vi "Fetch Device Info.vi"(8 "error in (no error)":errorcluster, 11 "Toggle 8 in":refnum<class "Toggle 8.lvclass">) -> (0 "error out":errorcluster, 2 "Device Info":string[][](array[string]), 3 "Toggle 8 out":refnum<class "Toggle 8.lvclass">)   [LabVIEW 2020, in "Toggle 8.lvclass"]
uses:
  Toggle 8.lvclass
  PIC-device/PIC-Device.lvclass
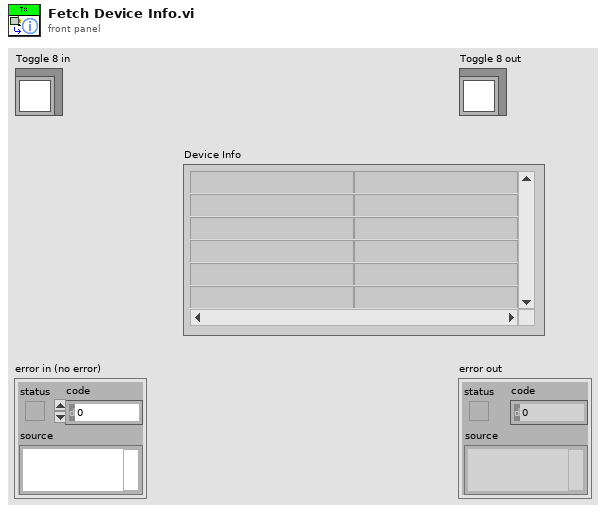
[diagram p1: front panel]
types:
  T1 = typedef "PIC-Device.lvclass/Register to Write.ctl" = cluster{"Register":u32, "Value":u32, "Dev Address":u32, "Physical Adress":u32}
  T2 = typedef "Device.lvclass/Device Information Cluster.ctl" = cluster{"Device Info":string[][], "Default Values":T1[], "Fetched info":string[][]}
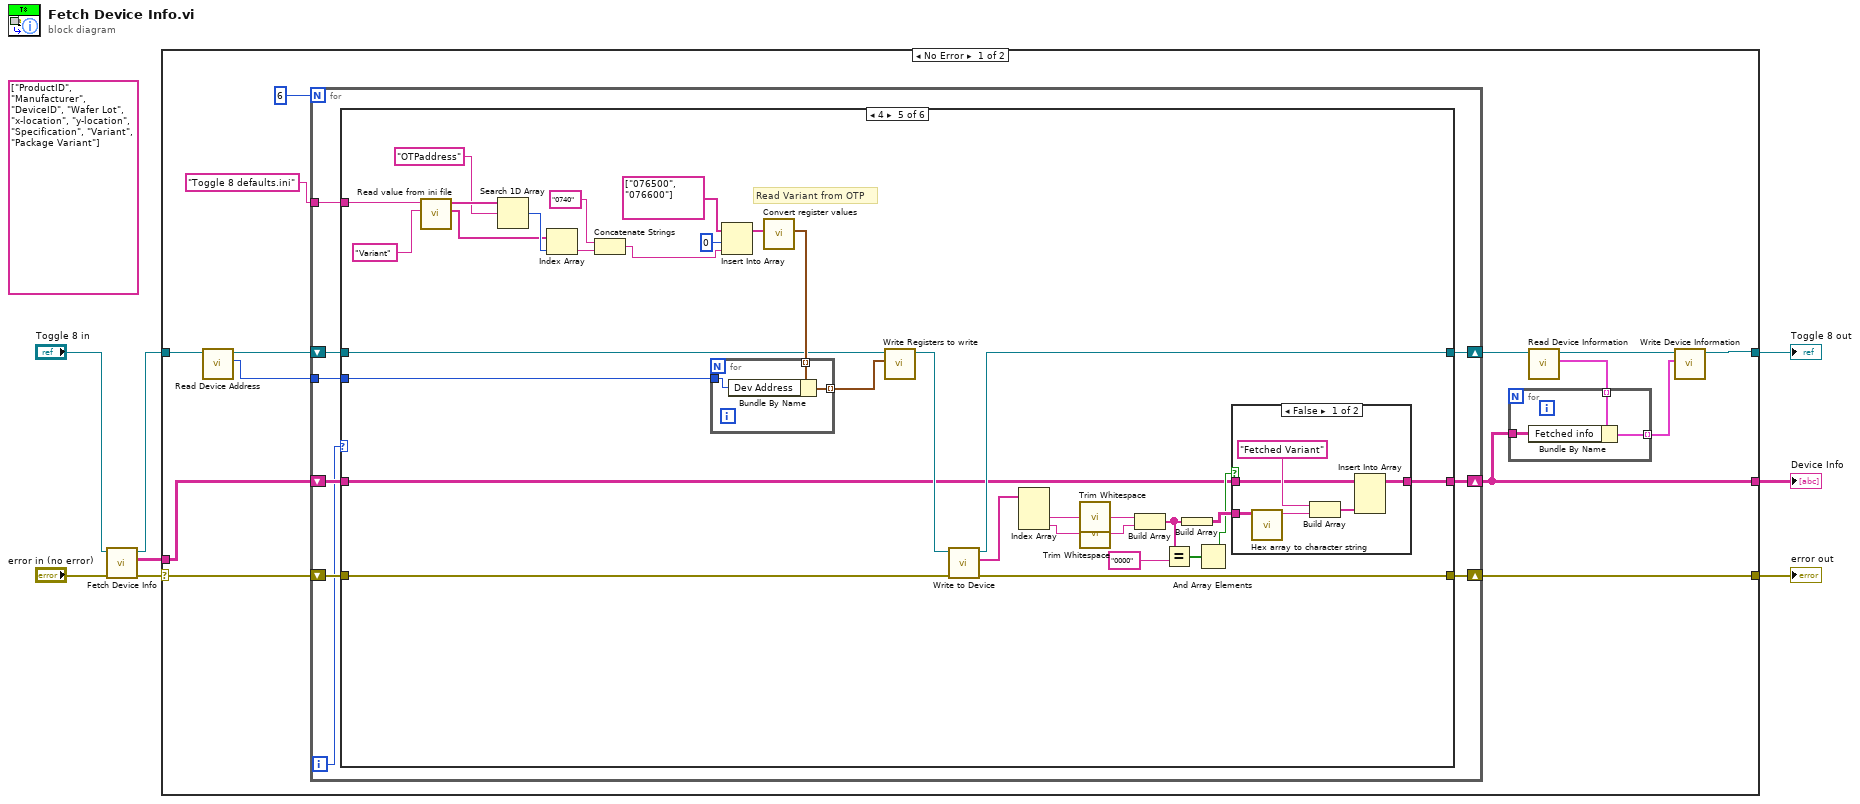
[diagram p0: block diagram]
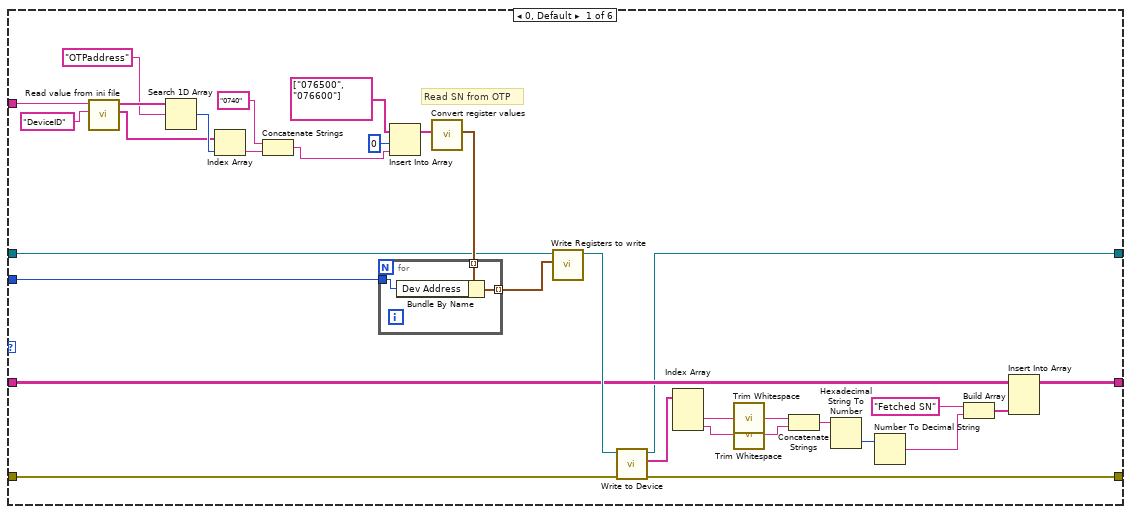
[diagram p2: hidden frame]
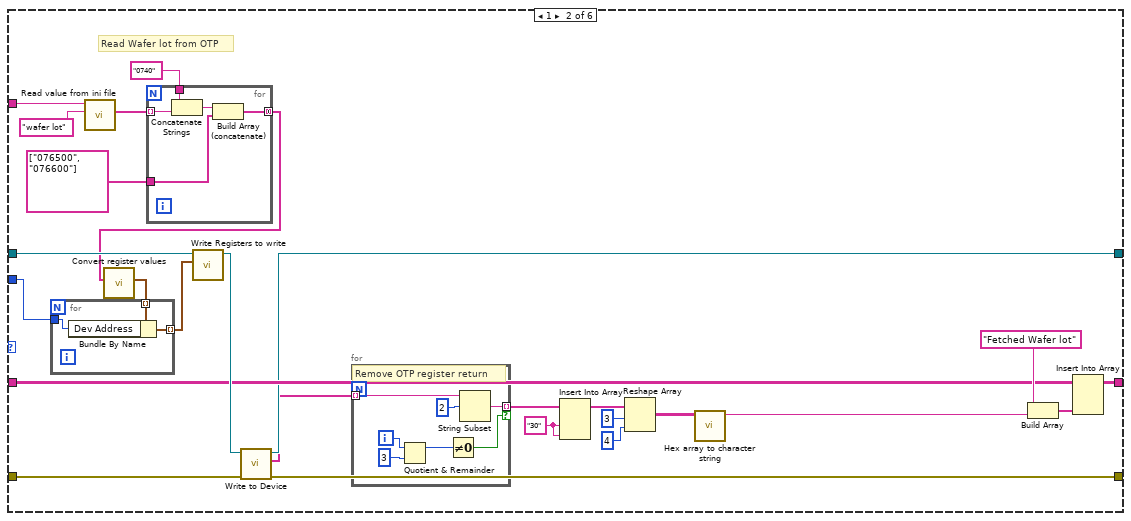
[diagram p3: hidden frame]
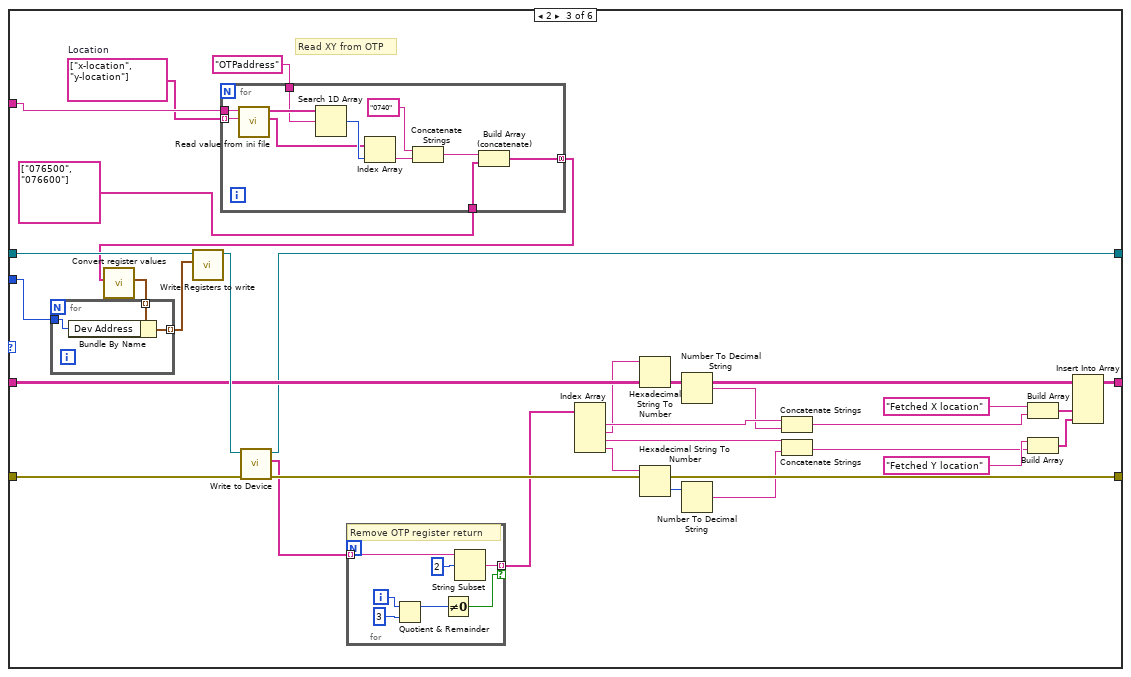
[diagram p4: hidden frame]
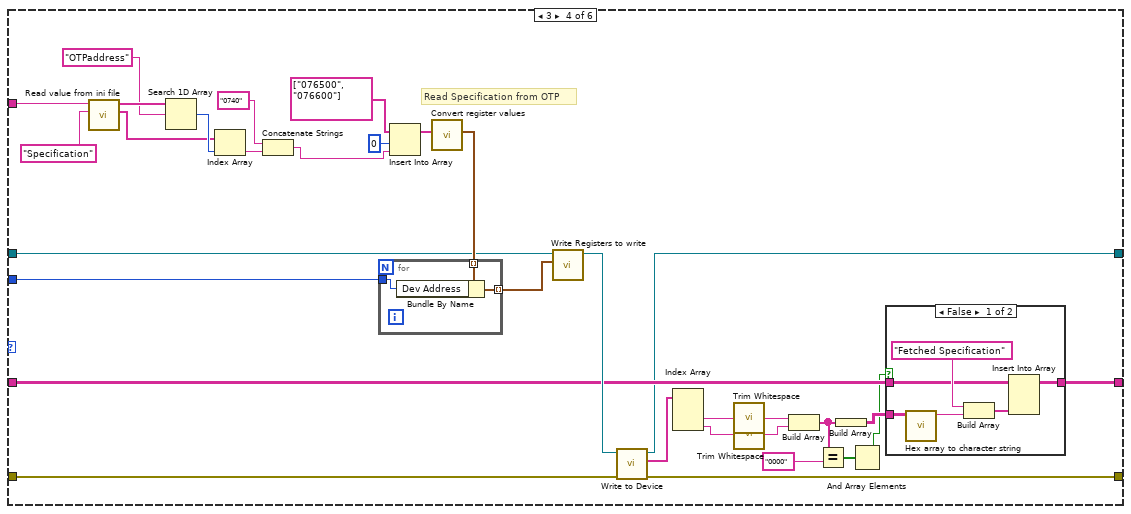
[diagram p5: hidden frame]
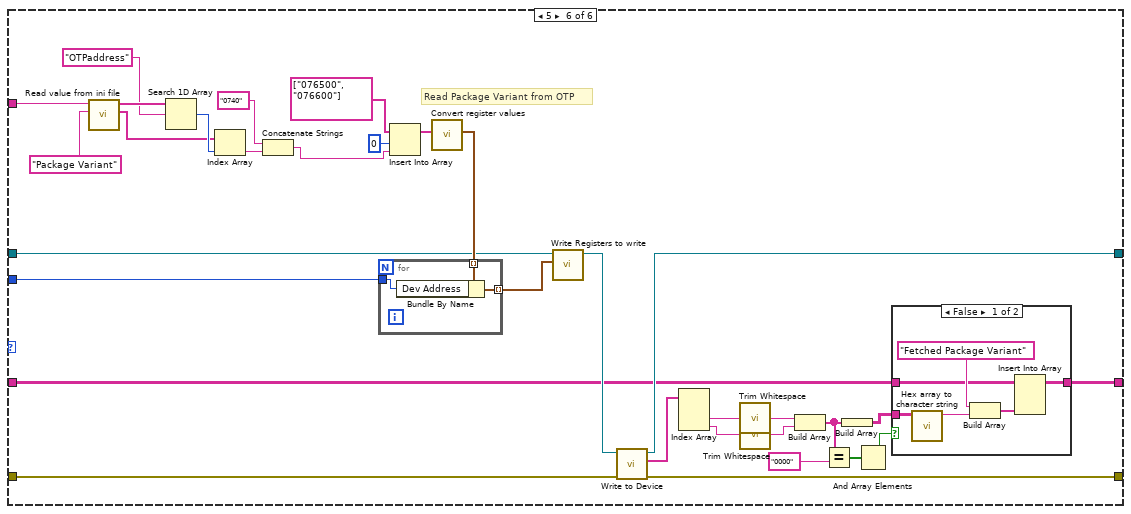
[diagram p8: hidden frame]
diagram:
  (unwired) string[] ["ProductID", "Manufacturer", "DeviceID", "Wafer Lot", "x-location", "y-location", "Specification", "Variant", "Package Variant"]
  n1 = call-parent "Fetch Device Info.vi"("error in (no error)"="error in (no error)", "PIC-Device in"="Toggle 8 in") -> ("error out"=w5:errorcluster, "Device Info"=w2:string[][], "PIC-Device out"=w3:refnum<class "Toggle 8.lvclass">)  [unwired: 7 in]
  n2 = case shown="No Error" w5 {
    selector: w5 -> [w22 w291]
    tunnel: [w20 w291] -> w8
    tunnel: [w14 w290] -> w7
    tunnel: w3 -> [w19 w290]
    tunnel: w2 -> [w21 w289]
    tunnel: [w13 w289] -> w1
    frame No Error {
      n3 = call-dynamic "Read Device Address.vi"("PIC-Device in"=w19) -> ("Device Address"=w12:u8, "PIC-Device out"=w11:refnum<class "Toggle 8.lvclass">)  [unwired: 9 in]
      n4 = for {
        N: 6 -> [_]
        tunnel: w12 -> [w26]
        shift-right: [w29] -> w20
        shift-left: w22 -> [w31]
        shift-right: [w28] -> w15
        shift-left: w11 -> [w25]
        shift-right: [w27] -> w13
        shift-left: w21 -> [w30]
        tunnel: "Toggle 8 defaults.ini" ("Ini file name") -> [w23]
        i -> [w24]
        n5 = case shown="4" w24 {
          tunnel: w31 -> [w62 w91 w137 w190 w232 w274]
          tunnel: w30 -> [w52 w89 w135 w185 w203 w246]
          tunnel: [w50 w87 w133 w184 w205 w244] -> w29
          tunnel: [w47 w84 w130 w181 w229 w271] -> w28
          tunnel: [w46 w83 w129 w180 w202 w247] -> w27
          tunnel: w26 -> [w45 w82 w128 w179 w228 w270]
          tunnel: w25 -> [w44 w81 w127 w178 w227 w269]
          tunnel: w23 -> [w42 w71 w111 w176 w225 w267]
          frame 0, Default {
            # "Read SN from OTP"
            n6 = call "Read value from ini file.vi"("Section"="DeviceID", "Ini file name"=w42) -> ("Values"=w37:string[], "Key names"=w40:string[])  [unwired: 8 in]
            n7 = Search 1D Array(1D array=w40, element="OTPaddress" ("String")) -> (index of element=w38:i32)  [unwired: 1 in]
            n8 = Index Array(array=w37, index=w38) -> (element=w36:string)
            n9 = Concatenate Strings("0740" ("Reg2read"), w36) -> (w34:string)
            n10 = Insert Into Array(array=string[] ["076500", "076600"], index=0, new element=w34) -> (w33:string[])
            n11 = call "Convert register values.vi"("Register strings"=w33) -> ("Register clusters out"=w49:T1[])  [unwired: 9 in, 1 out]
            n12 = for {
              tunnel: w49 -> [w66] mode=indexing
              tunnel: [w65] -> w48 mode=indexing
              tunnel: w45 -> [w64]
              n13 = Bundle By Name(cluster=w66, "Dev Address"=w64) -> (w65:T1)
            }
            n14 = call-dynamic "Write Registers to write.vi"("Registers to write"=w48, "Device in"=w44) -> ("Device out"=w63:refnum<class "Toggle 8.lvclass">)  [unwired: 9 in]
            n15 = call-dynamic "Write to Device.vi"("error in (no error)"=w62, "Device in"=w63) -> ("error out"=w50:errorcluster, "Return"=w57:string[], "Device out"=w47:refnum<class "Toggle 8.lvclass">)  [unwired: 7 in]
            n16 = Index Array(array=w57) -> (element #2=w56:string, element #3=w55:string)  [unwired: 3 in, 1 out]
            n17 = call <vilib>:"Trim Whitespace.vi"("string"=w56) -> ("trimmed string"=w58:string)  [unwired: 1 in]
            n18 = call <vilib>:"Trim Whitespace.vi"("string"=w55) -> ("trimmed string"=w59:string)  [unwired: 1 in]
            n19 = Concatenate Strings(w58, w59) -> (w61:string)
            n20 = Hexadecimal String To Number(string=w61) -> (number=w60:u32)  [unwired: 2 in, 1 out]
            n21 = Number To Decimal String(number=w60) -> (decimal integer string=w53:string)  [unwired: 1 in]
            n22 = Build Array("Fetched SN", w53) -> (w51:string[])
            n23 = Insert Into Array(array=w52, new element=w51) -> (w46:string[][])  [unwired: 2 in]
          }
          frame 1 {
            w78 = "30" ("new element/subarray")
            # "Read Wafer lot from OTP"
            n24 = call "Read value from ini file.vi"("Section"="wafer lot", "Ini file name"=w71) -> ("Values"=w70:string[])  [unwired: 8 in, 1 out]
            n25 = for {
              tunnel: string[] ["076500", "076600"] -> [w94]
              tunnel: [w93] -> w73 mode=concatenating
              tunnel: w70 -> [w97] mode=indexing
              tunnel: "0740" ("Reg2read") -> [w96]
              n26 = Concatenate Strings(w96, w97) -> (w95:string)
              n27 = Build Array (concatenate)(w95, w94) -> (w93:string[])
            }
            n28 = call "Convert register values.vi"("Register strings"=w73) -> ("Register clusters out"=w86:T1[])  [unwired: 9 in, 1 out]
            n29 = for {
              tunnel: w86 -> [w107] mode=indexing
              tunnel: [w106] -> w85 mode=indexing
              tunnel: w82 -> [w105]
              n30 = Bundle By Name(cluster=w107, "Dev Address"=w105) -> (w106:T1)
            }
            n31 = call-dynamic "Write Registers to write.vi"("Registers to write"=w85, "Device in"=w81) -> ("Device out"=w92:refnum<class "Toggle 8.lvclass">)  [unwired: 9 in]
            n32 = call-dynamic "Write to Device.vi"("error in (no error)"=w91, "Device in"=w92) -> ("error out"=w87:errorcluster, "Return"=w75:string[], "Device out"=w84:refnum<class "Toggle 8.lvclass">)  [unwired: 7 in]
            n33 = for {
              tunnel: w75 -> [w104] mode=indexing
              tunnel: [w102] -> w79 mode=indexing if=w98
              i -> [w101]
              # "Remove OTP register return"
              n34 = Quotient & Remainder(x=w101, y=3) -> (x-y*floor(x/y)=w99:i32)  [unwired: 1 out]
              n35 = Not Equal To 0?(x=w99) -> (x != 0?=w98:bool)
              n36 = String Subset(string=w104, offset (0)=2) -> (substring=w102:string)  [unwired: 1 in]
            }
            n37 = Insert Into Array(array=w79, new element #1=w78, new element #2=w78) -> (w80:string[])  [unwired: 1 in]
            n38 = Reshape Array(w80, 3 ("dimension size"), 4 ("dimension size")) -> (w68:string[][])
            n39 = call "Hex array to character string.vi"("Array"=w68) -> ("String"=w67:string)  [unwired: 10 in]
            n40 = Build Array("Fetched Wafer lot", w67) -> (w88:string[])
            n41 = Insert Into Array(array=w89, new element=w88) -> (w83:string[][])  [unwired: 2 in]
          }
          frame 2 {
            w110 = string[] ["x-location", "y-location"]  # Location
            # "Read XY from OTP"
            n42 = for {
              tunnel: "OTPaddress" ("String") -> [w147]
              tunnel: w111 -> [w143]
              tunnel: w110 -> [w142] mode=indexing
              tunnel: string[] ["076500", "076600"] -> [w140]
              tunnel: [w139] -> w108 mode=concatenating
              n43 = call "Read value from ini file.vi"("Section"=w142, "Ini file name"=w143) -> ("Values"=w145:string[], "Key names"=w148:string[])  [unwired: 8 in]
              n44 = Search 1D Array(1D array=w148, element=w147) -> (index of element=w146:i32)  [unwired: 1 in]
              n45 = Index Array(array=w145, index=w146) -> (element=w144:string)
              n46 = Concatenate Strings("0740" ("Reg2read"), w144) -> (w141:string)
              n47 = Build Array (concatenate)(w141, w140) -> (w139:string[])
            }
            n48 = call "Convert register values.vi"("Register strings"=w108) -> ("Register clusters out"=w132:T1[])  [unwired: 9 in, 1 out]
            n49 = for {
              tunnel: w132 -> [w159] mode=indexing
              tunnel: [w158] -> w131 mode=indexing
              tunnel: w128 -> [w157]
              n50 = Bundle By Name(cluster=w159, "Dev Address"=w157) -> (w158:T1)
            }
            n51 = call-dynamic "Write Registers to write.vi"("Registers to write"=w131, "Device in"=w127) -> ("Device out"=w138:refnum<class "Toggle 8.lvclass">)  [unwired: 9 in]
            n52 = call-dynamic "Write to Device.vi"("error in (no error)"=w137, "Device in"=w138) -> ("error out"=w133:errorcluster, "Return"=w126:string[], "Device out"=w130:refnum<class "Toggle 8.lvclass">)  [unwired: 7 in]
            n53 = for {
              tunnel: w126 -> [w156] mode=indexing
              tunnel: [w154] -> w125 mode=indexing if=w150
              i -> [w153]
              # "Remove OTP register return"
              n54 = Quotient & Remainder(x=w153, y=3) -> (x-y*floor(x/y)=w151:i32)  [unwired: 1 out]
              n55 = Not Equal To 0?(x=w151) -> (x != 0?=w150:bool)
              n56 = String Subset(string=w156, offset (0)=2) -> (substring=w154:string)  [unwired: 1 in]
            }
            n57 = Index Array(array=w125) -> (element #1=w124:string, element #2=w114:string, element #3=w122:string, element #4=w117:string)  [unwired: 4 in]
            n58 = Hexadecimal String To Number(string=w114) -> (number=w115:u32)  [unwired: 2 in, 1 out]
            n59 = Hexadecimal String To Number(string=w117) -> (number=w118:u32)  [unwired: 2 in, 1 out]
            n60 = Number To Decimal String(number=w115) -> (decimal integer string=w113:string)  [unwired: 1 in]
            n61 = Number To Decimal String(number=w118) -> (decimal integer string=w116:string)  [unwired: 1 in]
            n62 = Concatenate Strings(w124, w113) -> (w123:string)
            n63 = Concatenate Strings(w122, w116) -> (w120:string)
            n64 = Build Array("Fetched X location", w123) -> (w134:string[])
            n65 = Build Array("Fetched Y location", w120) -> (w119:string[])
            n66 = Insert Into Array(array=w135, new element #1=w134, new element #2=w119) -> (w129:string[][])  [unwired: 2 in]
          }
          frame 3 {
            # "Read Specification from OTP"
            n67 = call "Read value from ini file.vi"("Section"="Specification", "Ini file name"=w176) -> ("Values"=w171:string[], "Key names"=w174:string[])  [unwired: 8 in]
            n68 = Search 1D Array(1D array=w174, element="OTPaddress" ("String")) -> (index of element=w172:i32)  [unwired: 1 in]
            n69 = Index Array(array=w171, index=w172) -> (element=w170:string)
            n70 = Concatenate Strings("0740" ("Reg2read"), w170) -> (w168:string)
            n71 = Insert Into Array(array=string[] ["076500", "076600"], index=0, new element=w168) -> (w167:string[])
            n72 = call "Convert register values.vi"("Register strings"=w167) -> ("Register clusters out"=w183:T1[])  [unwired: 9 in, 1 out]
            n73 = for {
              tunnel: w183 -> [w201] mode=indexing
              tunnel: [w200] -> w182 mode=indexing
              tunnel: w179 -> [w199]
              n74 = Bundle By Name(cluster=w201, "Dev Address"=w199) -> (w200:T1)
            }
            n75 = call-dynamic "Write Registers to write.vi"("Registers to write"=w182, "Device in"=w178) -> ("Device out"=w191:refnum<class "Toggle 8.lvclass">)  [unwired: 9 in]
            n76 = call-dynamic "Write to Device.vi"("error in (no error)"=w190, "Device in"=w191) -> ("error out"=w184:errorcluster, "Return"=w187:string[], "Device out"=w181:refnum<class "Toggle 8.lvclass">)  [unwired: 7 in]
            n77 = Index Array(array=w187) -> (element #2=w186:string, element #3=w164:string)  [unwired: 3 in, 1 out]
            n78 = call <vilib>:"Trim Whitespace.vi"("string"=w186) -> ("trimmed string"=w188:string)  [unwired: 1 in]
            n79 = call <vilib>:"Trim Whitespace.vi"("string"=w164) -> ("trimmed string"=w189:string)  [unwired: 1 in]
            n80 = Build Array(w188, w189) -> (w163:string[])
            n81 = Equal?(x=w163, y="0000") -> (x = y?=w161:bool[])
            n82 = Build Array(w163) -> (w165:string[][])
            n83 = And Array Elements(Boolean array=w161) -> (logical AND=w160:bool)
            n84 = case shown="False" w160 {
              tunnel: w185 -> [w196 w198]
              tunnel: [w194 w198] -> w180
              tunnel: w165 -> [w192 _]
              frame False {
                n85 = call "Hex array to character string.vi"("Array"=w192) -> ("String"=w193:string)  [unwired: 10 in]
                n86 = Build Array("Fetched Specification", w193) -> (w195:string[])
                n87 = Insert Into Array(array=w196, new element=w195) -> (w194:string[][])  [unwired: 2 in]
              }
              frame True {
              }
            }
          }
          frame 4 {
            # "Read Variant from OTP"
            n88 = call "Read value from ini file.vi"("Section"="Variant", "Ini file name"=w225) -> ("Values"=w220:string[], "Key names"=w223:string[])  [unwired: 8 in]
            n89 = Search 1D Array(1D array=w223, element="OTPaddress" ("String")) -> (index of element=w221:i32)  [unwired: 1 in]
            n90 = Index Array(array=w220, index=w221) -> (element=w219:string)
            n91 = Concatenate Strings("0740" ("Reg2read"), w219) -> (w217:string)
            n92 = Insert Into Array(array=string[] ["076500", "076600"], index=0, new element=w217) -> (w216:string[])
            n93 = call "Convert register values.vi"("Register strings"=w216) -> ("Register clusters out"=w231:T1[])  [unwired: 9 in, 1 out]
            n94 = for {
              tunnel: w231 -> [w243] mode=indexing
              tunnel: [w242] -> w230 mode=indexing
              tunnel: w228 -> [w241]
              n95 = Bundle By Name(cluster=w243, "Dev Address"=w241) -> (w242:T1)
            }
            n96 = call-dynamic "Write Registers to write.vi"("Registers to write"=w230, "Device in"=w227) -> ("Device out"=w233:refnum<class "Toggle 8.lvclass">)  [unwired: 9 in]
            n97 = call-dynamic "Write to Device.vi"("error in (no error)"=w232, "Device in"=w233) -> ("error out"=w205:errorcluster, "Return"=w204:string[], "Device out"=w229:refnum<class "Toggle 8.lvclass">)  [unwired: 7 in]
            n98 = Index Array(array=w204) -> (element #2=w212:string, element #3=w210:string)  [unwired: 3 in, 1 out]
            n99 = call <vilib>:"Trim Whitespace.vi"("string"=w212) -> ("trimmed string"=w213:string)  [unwired: 1 in]
            n100 = call <vilib>:"Trim Whitespace.vi"("string"=w210) -> ("trimmed string"=w214:string)  [unwired: 1 in]
            n101 = Build Array(w213, w214) -> (w209:string[])
            n102 = Equal?(x=w209, y="0000") -> (x = y?=w207:bool[])
            n103 = Build Array(w209) -> (w211:string[][])
            n104 = And Array Elements(Boolean array=w207) -> (logical AND=w206:bool)
            n105 = case shown="False" w206 {
              tunnel: w203 -> [w238 w240]
              tunnel: [w236 w240] -> w202
              tunnel: w211 -> [w234 _]
              frame False {
                n106 = call "Hex array to character string.vi"("Array"=w234) -> ("String"=w235:string)  [unwired: 10 in]
                n107 = Build Array("Fetched Variant", w235) -> (w237:string[])
                n108 = Insert Into Array(array=w238, new element=w237) -> (w236:string[][])  [unwired: 2 in]
              }
              frame True {
              }
            }
          }
          frame 5 {
            # "Read Package Variant from OTP"
            n109 = call "Read value from ini file.vi"("Section"="Package Variant", "Ini file name"=w267) -> ("Values"=w262:string[], "Key names"=w265:string[])  [unwired: 8 in]
            n110 = Search 1D Array(1D array=w265, element="OTPaddress" ("String")) -> (index of element=w263:i32)  [unwired: 1 in]
            n111 = Index Array(array=w262, index=w263) -> (element=w261:string)
            n112 = Concatenate Strings("0740" ("Reg2read"), w261) -> (w259:string)
            n113 = Insert Into Array(array=string[] ["076500", "076600"], index=0, new element=w259) -> (w258:string[])
            n114 = call "Convert register values.vi"("Register strings"=w258) -> ("Register clusters out"=w273:T1[])  [unwired: 9 in, 1 out]
            n115 = for {
              tunnel: w273 -> [w285] mode=indexing
              tunnel: [w284] -> w272 mode=indexing
              tunnel: w270 -> [w283]
              n116 = Bundle By Name(cluster=w285, "Dev Address"=w283) -> (w284:T1)
            }
            n117 = call-dynamic "Write Registers to write.vi"("Registers to write"=w272, "Device in"=w269) -> ("Device out"=w275:refnum<class "Toggle 8.lvclass">)  [unwired: 9 in]
            n118 = call-dynamic "Write to Device.vi"("error in (no error)"=w274, "Device in"=w275) -> ("error out"=w244:errorcluster, "Return"=w245:string[], "Device out"=w271:refnum<class "Toggle 8.lvclass">)  [unwired: 7 in]
            n119 = Index Array(array=w245) -> (element #2=w254:string, element #3=w252:string)  [unwired: 3 in, 1 out]
            n120 = call <vilib>:"Trim Whitespace.vi"("string"=w254) -> ("trimmed string"=w255:string)  [unwired: 1 in]
            n121 = call <vilib>:"Trim Whitespace.vi"("string"=w252) -> ("trimmed string"=w256:string)  [unwired: 1 in]
            n122 = Build Array(w255, w256) -> (w251:string[])
            n123 = Equal?(x=w251, y="0000") -> (x = y?=w249:bool[])
            n124 = Build Array(w251) -> (w253:string[][])
            n125 = And Array Elements(Boolean array=w249) -> (logical AND=w248:bool)
            n126 = case shown="False" w248 {
              tunnel: w246 -> [w280 w282]
              tunnel: [w278 w282] -> w247
              tunnel: w253 -> [w276 _]
              frame False {
                n127 = call "Hex array to character string.vi"("Array"=w276) -> ("String"=w277:string)  [unwired: 10 in]
                n128 = Build Array("Fetched Package Variant", w277) -> (w279:string[])
                n129 = Insert Into Array(array=w280, new element=w279) -> (w278:string[][])  [unwired: 2 in]
              }
              frame True {
              }
            }
          }
        }
      }
      n130 = call-dynamic "Read Device Information.vi"("Device in"=w15) -> ("Device Info"=w18:T2[], "Device out"=w16:refnum<class "Toggle 8.lvclass">)  [unwired: 8 in, 1 out]
      n131 = for {
        tunnel: w18 -> [w288] mode=indexing
        tunnel: w13 -> [w286]
        tunnel: [w287] -> w17 mode=indexing
        n132 = Bundle By Name(cluster=w288, "Fetched info"=w286) -> (w287:T2)
      }
      n133 = call-dynamic "Write Device Information.vi"("Device Info"=w17, "Device in"=w16) -> ("Device out"=w14:refnum<class "Toggle 8.lvclass">)  [unwired: 8 in, 1 out]
    }
    frame Error {
    }
  }
  "error out" <- w8
  "Toggle 8 out" <- w7
  "Device Info" <- w1
